vi "User-Defined Comparison.vi"(1 "Expected Value":variant, 2 "Resulting Value":variant) -> (0 "Comparison Result":bool)   [LabVIEW 2023]
doc: "This is an example of a user-defined comparison VI, which uses the <B>Greater or Equal</B> function to compare the resulting value with the expected value. \nYou can specify the comparison type by changing a comparison function on the block diagram. Do not change the controls and connector pane pattern."
panel:
  # "Overview:  This is an example of a user-defined comparison VI, which uses the Greater or Equal function to compare the resulting value with the expected value.\nRequirements: LabVIEW Full Development System, Unit Test Framework Toolkit\nInstructions:  You can specify the comparison type by changing a comparison function on the block diagram. Do not change the controls and connector pane pattern."
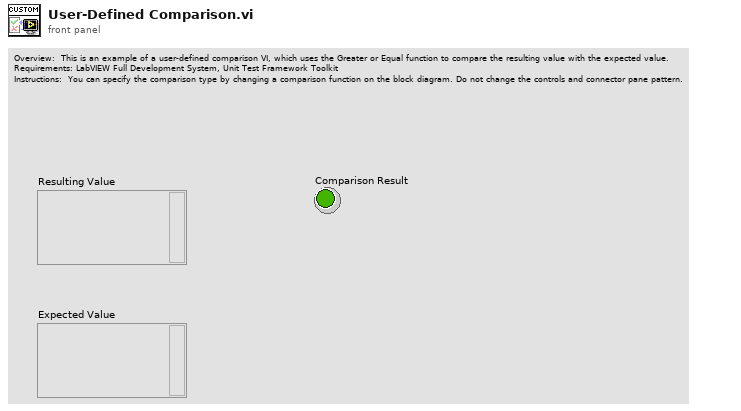
[diagram p1: front panel]
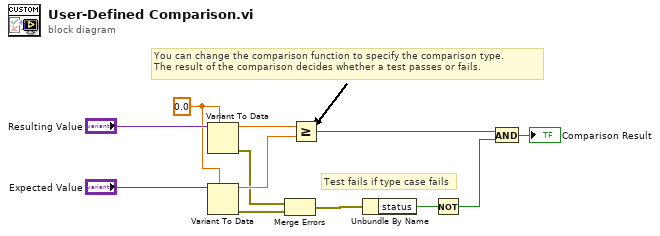
[diagram p0: block diagram]
diagram:
  w9 = 0.0
  # "You can change the comparison function to specify the comparison type.\nThe result of the comparison decides whether a test passes or fails."
  # "Test fails if type case fails"
  n1 = Variant To Data(type=w9, Variant="Resulting Value") -> (data=w11:dbl, error out=w7:errorcluster)  [unwired: 1 in]
  n2 = Variant To Data(type=w9, Variant="Expected Value") -> (data=w8:dbl, error out=w6:errorcluster)  [unwired: 1 in]
  n3 = Merge Errors(w7, w6) -> (w4:errorcluster)
  n4 = Greater Or Equal?(x=w11, y=w8) -> (x >= y?=w5:bool)
  n5 = Unbundle By Name(w4) -> ("status"=w3:bool)
  n6 = Not(x=w3) -> (.not. x?=w2:bool)
  n7 = And(x=w5, y=w2) -> (x .and. y?=→"Comparison Result":bool)
